vi "TS Run Start.vi"(8 "error in (no error)":errorcluster, 11 "Water Tunnel Test Stand in":refnum<class "Water Tunnel Test Stand.lvclass">) -> (0 "error out":errorcluster, 3 "Water Tunnel Test Stand out":refnum<class "Water Tunnel Test Stand.lvclass">)   [LabVIEW 2019, in "Test Stands.lvlib" / "Water Tunnel Test Stand.lvclass"]
uses:
  Water Tunnel Test Stand.lvclass
  Results/Results Method.ctl
  Results/Results.lvlib
  Generic Test Stand/Generic Test Stand.lvclass
  Results/Water Tunnel Results/Water Tunnel Results.lvclass
  C:/Users/wg/Documents/LV_Projects/test-stand/App/Generic Test Stand/Generic Test Stand.lvclass
  C:/Users/wg/Documents/LV_Projects/test-stand/App/Results/Results.lvclass
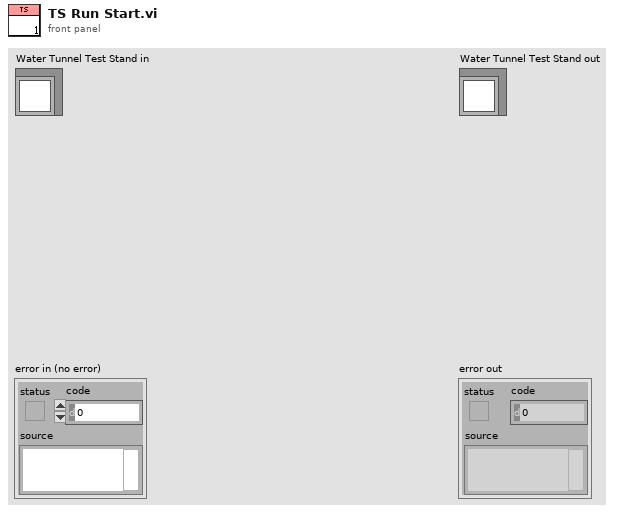
[diagram p1: front panel]
types:
  T1 = typedef "Results.lvlib/Results Method.ctl" = enum16{"Get", "Set"}
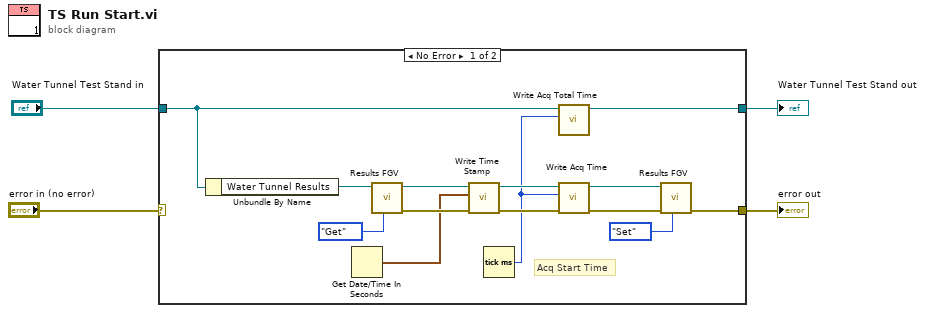
[diagram p0: block diagram]
diagram:
  n1 = case shown="No Error" "error in (no error)" {
    selector: "error in (no error)" -> [_ w20]
    tunnel: [w9 w20] -> w4
    tunnel: [w6 w19] -> w3
    tunnel: "Water Tunnel Test Stand in" -> [w7 w19]
    frame No Error {
      # "Acq Start Time"
      n2 = Unbundle By Name(w7) -> ("Water Tunnel Results"=w15:refnum<class "Water Tunnel Results.lvclass">)
      n3 = Get Date/Time In Seconds() -> (seconds since 1Jan1904=w8:timestamp)
      n4 = call-dynamic "Results FGV.vi"("Method"=Results_Method."Get", "Water Tunnel Results in"=w15) -> ("error out"=w12:errorcluster, "Water Tunnel  Results out"=w13:refnum<class "Water Tunnel Results.lvclass">)  [unwired: 8 in]
      n5 = call-dynamic "Write Time Stamp.vi"("error in (no error)"=w12, "Time Stamp"=w8, "Results in"=w13) -> ("error out"=w11:errorcluster, "Results out"=w18:refnum<class "Water Tunnel Results.lvclass">)  [unwired: 7 in]
      n6 = Tick Count (ms)() -> (millisecond timer value=w5:u32)
      n7 = call "Write Acq Total Time.vi"("Acq Total Time"=w5, "Generic Test Stand in"=w7) -> ("Generic Test Stand out"=w6:refnum<class "Water Tunnel Test Stand.lvclass">)  [unwired: 8 in, 1 out]
      n8 = call "Write Acq Time.vi"("error in (no error)"=w11, "Acq Time"=w5, "Results in"=w18) -> ("error out"=w10:errorcluster, "Results out"=w17:refnum<class "Water Tunnel Results.lvclass">)  [unwired: 7 in]
      n9 = call-dynamic "Results FGV.vi"("Method"=Results_Method."Set", "error in"=w10, "Water Tunnel Results in"=w17) -> ("error out"=w9:errorcluster)  [unwired: 7 in, 1 out]
    }
    frame Error {
    }
  }
  "error out" <- w4
  "Water Tunnel Test Stand out" <- w3
